vi "arm pid.vi"(1 "Setpoint":dbl) -> (0 "Output":dbl)   [LabVIEW 2014]
uses:
  typedefs/safety data/container arm safety data.ctl
  global variables/devrefs.vi
  <vilib>/addons/control/pid/pid.llb/PID (DBL).vi
  global variables/safeties.vi
  <vilib>/addons/control/pid/NI_PID_pid.lvlib
panel:
  out "Waveform Chart":dbl(graph)
  out "Distance":dbl
  out "output cluster":T1
  in  "PID gains":T2={"proportional gain (Kc)"=0.045, "integral time (Ti, min)"=0.0075, "derivative time (Td, min)"=0.00085}
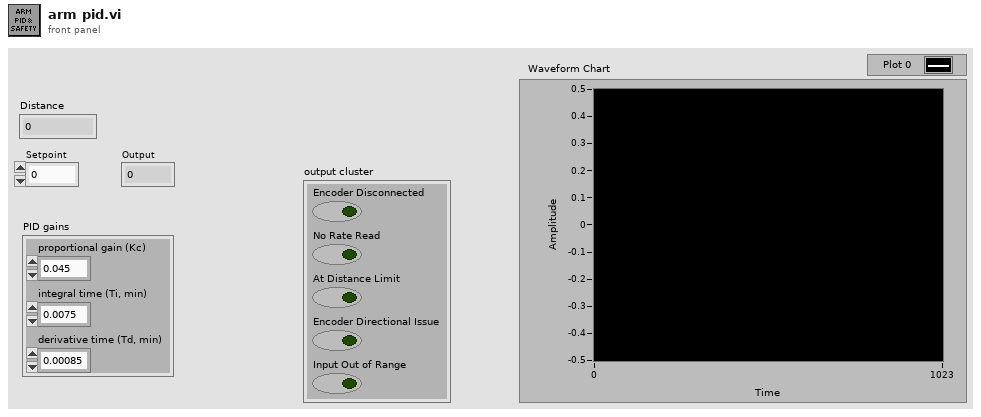
[diagram p1: front panel]
types:
  T1 = typedef "container arm safety data.ctl" = cluster{"Encoder Disconnected":bool, "No Rate Read":bool, "At Distance Limit":bool, "Encoder Directional Issue":bool, "Input Out of Range":bool}
  T2 = cluster{"proportional gain (Kc)":dbl, "integral time (Ti, min)":dbl, "derivative time (Td, min)":dbl}
  T3 = typedef "subStates.ctl" = enum16{"null", "wait", "driver control", "auto", "manual override", "hold position", "rotate", "test", "end"}
  T4 = typedef "WPI_EncoderDevRef.ctl" = cluster{"DevStatus":errorcluster, "EncoderIndex":T5, "CounterIndex":T6, "DistancePerCount":dbl, "Decoding Type":T7}
  T5 = typedef "FPGA_EncoderIdx.ctl" = enum8{"Enc 0", "Enc 1", "Enc 2", "Enc 3", "Enc 4", "Enc 5", "Enc 6", "Enc 7", "Invalid"}
  T6 = typedef "FPGA_CounterCtrSystemIndex.ctl" = enum8{"Ctr 0", "Ctr 1", "Ctr 2", "Ctr 3", "Ctr 4", "Ctr 5", "Ctr 6", "Ctr 7", "Invalid"}
  T7 = typedef "WPI_EncoderType.ctl" = enum16{"1x", "2x", "4x"}
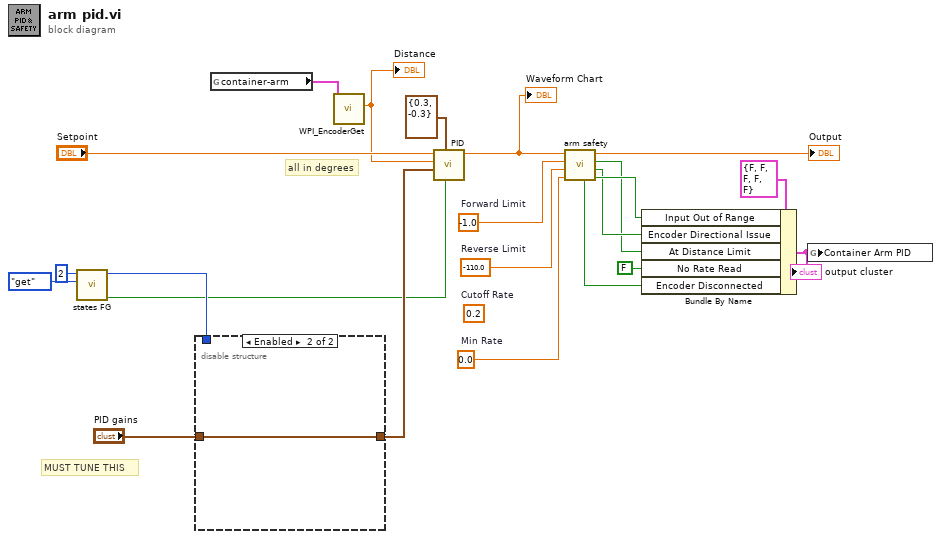
[diagram p0: block diagram]
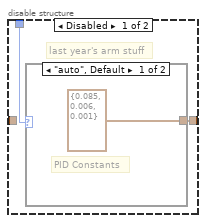
[diagram p2: hidden frame]
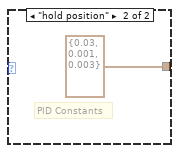
[diagram p3: hidden frame]
diagram:
  w7 = 0.0  # Min Rate
  (unwired) 0.2  # Cutoff Rate
  w8 = -110.0  # Reverse Limit
  w9 = -1.0  # Forward Limit
  # "MUST TUNE THIS"
  # "all in degrees"
  n1 = call "states FG.vi"("menu (get)"=enum16{"set", "get"}."get", "Loop ID"=2) -> ("first call?"=w15:bool, "subState out"=w16:T3)  [unwired: 6 in, 2 out]
  n2 = disable-structure shown="Enabled" {
    disable-tunnel: [w24 w27] -> w19
    disable-tunnel: w16 -> [w23 _]
    disable-tunnel: "PID gains" -> [_ w27]
    frame Disabled {
      # "last year's arm stuff"
      n3 = case shown="\"auto\", Default" w23 {
        tunnel: [T2 {"proportional gain (Kc)"=0.085, "integral time (Ti, min)"=0.006, "derivative time (Td, min)"=0.001} ("PID gains") T2 {"proportional gain (Kc)"=0.03, "integral time (Ti, min)"=0.001, "derivative time (Td, min)"=0.003} ("Hold Position PID gains")] -> w24
        frame "auto", Default {
          # "PID Constants"
        }
        frame "hold position" {
          # "PID Constants"
        }
      }
    }
    frame Enabled {
    }
  }
  n4 = global read "devrefs.vi" "container-arm"() -> (w14:T4)
  n5 = call <vilib>:"WPI_EncoderGet.vi"("EncoderDevRef"=w14) -> ("Distance"=w21:dbl)  [unwired: 5 in, 5 out]
  "Distance" <- w21
  n6 = call-poly <vilib>:"PID.vi"("reinitialize? (F)"=w15, "output range"=cluster{"output high":dbl, "output low":dbl} {"output high"=0.3, "output low"=-0.3}, "PID gains"=w19, "process variable"=w21, "setpoint"="Setpoint") -> ("output"=w1:dbl)  [unwired: 5 in, 1 out]
  "Waveform Chart" <- w1
  n7 = call "arm safety.vi"("Min Rate"=w7, "Reverse Limit"=w8, "Forward Limit"=w9, "Desired Rate"=w1) -> ("Input Out of Range"=w5:bool, "Encoder Directional Issue"=w4:bool, "At Distance Limit"=w3:bool, "Output Rate"=→"Output":dbl, "Encoder Failure"=w6:bool)  [unwired: 3 in]
  n8 = Bundle By Name(cluster=T1 {"Encoder Disconnected"=FALSE, "No Rate Read"=FALSE, "At Distance Limit"=FALSE, "Encoder Directional Issue"=FALSE, "Input Out of Range"=FALSE} ("Container Arm PID"), "Input Out of Range"=w5, "Encoder Directional Issue"=w4, "At Distance Limit"=w3, "No Rate Read"=FALSE, "Encoder Disconnected"=w6) -> (w11:T1)
  "output cluster" <- w11
  n9 = global write "safeties.vi" "Container Arm PID"(w11) -> ()
